vi "test.vi"() -> ()   [LabVIEW 2012]
uses:
  <vilib>/Platform/TimedLoop/XDataNode/timing_clust.ctl
  <vilib>/Platform/TimedLoop/XDataNode/nitl_modes.ctl
  <vilib>/Platform/TimedLoop/XDataNode/wakeup.ctl
  <vilib>/platform/TimedLoop/XDataNode/XDataNode.xnode
  <vilib>/Platform/TimedLoop/XDataNode/XDNodeRunTimeDep.lvlib
panel:
  out "CoolSnap Slave":bool
  out "Pixelfly Slave":bool
  out "ProEM Slave":bool
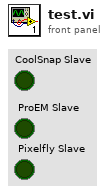
[diagram p1: front panel]
types:
  T1 = typedef "XDNodeRunTimeDep.lvlib/timing_clust.ctl" = cluster{"Expected End [f-1]":u64, "Actual End [f-1]":u64, "Finished Late? [f-1]":bool, "Expected End [i-1]":u64, "Actual End [i-1]":u64, "Finished Late? [i-1]":bool, "Expected Start [i]":u64, "Actual Start [i]":u64, "Expected Start [f]":u64, "Actual Start [f]":u64, "Source Name":string, "Structure Name":string, "Period":i64, "Deadline":i64, "Offset":i64, "Start":i64, "Priority":i32, "Timeout":i32, "Mode":T2, "Wakeup Reason":T3, "Error":errorcluster, "Source Type":string, "Secondary Source Type":string, "Global End Time":u64, "Global Start Time":u64, "Frame Duration":u64, "Iteration Duration":u64, "Assigned CPU":i32, "I/O Scan Engine Mode":u32}
  T2 = typedef "XDNodeRunTimeDep.lvlib/nitl_modes.ctl" = enum32{"No Change", "Process missed periods, maintain original phase", "Discard missed periods, maintain original phase", "Process missed periods, ignore original phase", "Discard missed periods, ignore original phase"}
  T3 = typedef "XDNodeRunTimeDep.lvlib/wakeup.ctl" = enum32{"Normal", "Aborted", "Asynchronous wakeup", "Timing source error", "Timed loop error", "Timeout"}
  T4 = typedef "LVDateTimeRec.ctl" = cluster{"fractional second":dbl, "second":i32, "minute":i32, "hour":i32, "day of month":i32, "month":i32, "year":i32, "day of week":i32, "day of year":i32, "DST":i32}
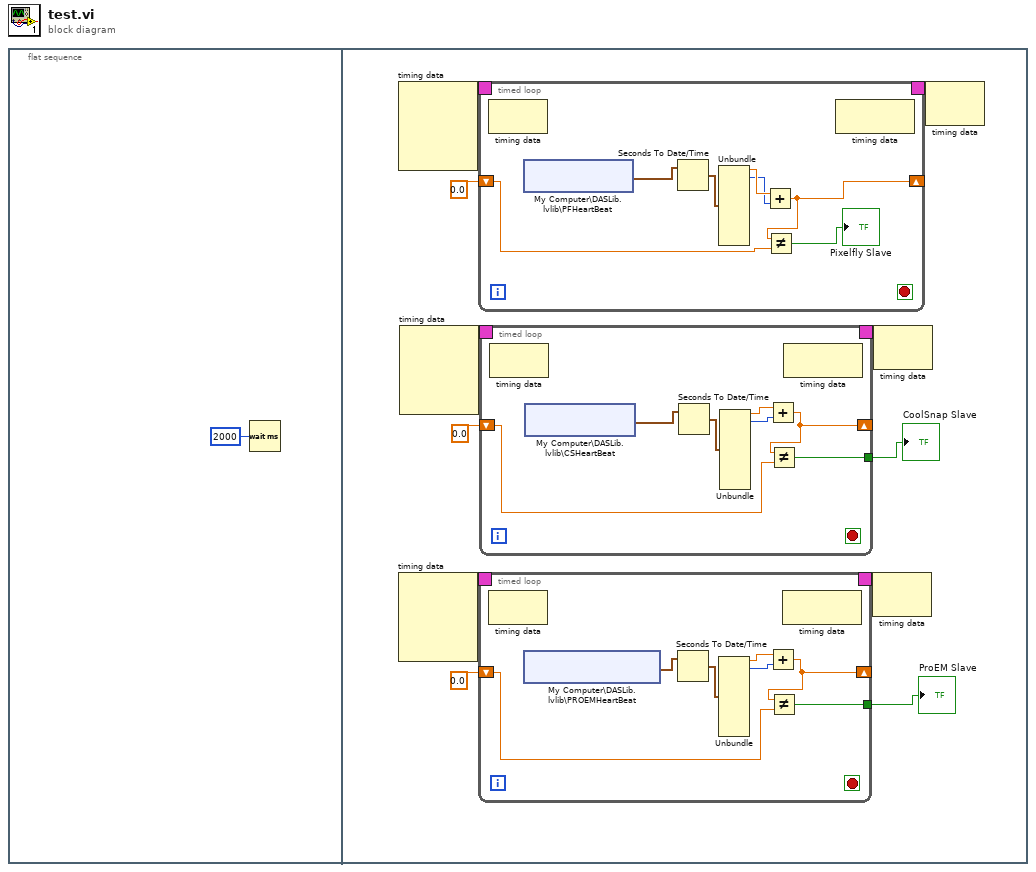
[diagram p0: block diagram]
diagram:
  n1 = flat-sequence {
    frame #0 {
      n2 = Wait (ms)(milliseconds to wait=u32 2000) -> ()  [unwired: 1 out]
    }
    frame #1 {
      n3 = node-c288() -> (w12:T1)  [unwired: 4 in]
      n4 = node-c288() -> (w8:T1)  [unwired: 4 in]
      n5 = node-c288() -> (w10:T1)  [unwired: 4 in]
      n6 = timed-loop {
        timing: w12 -> [_]
        timing-out: [_] -> w11
        shift-right: [w37] -> _
        shift-left: 0.0 ("fractional second") -> [w36]
        stop <- _ stop-if-true
        n7 = node-c288() -> ()  [unwired: 1 in, 1 out]
        n8 = shared-variable "My Computer\\DASLib.lvlib\\PFHeartBeat"() -> (w41:timestamp)  [unwired: 1 in, 2 out]
        n9 = Seconds To Date/Time(time stamp (now)=w41) -> (date time rec=w40:T4)  [unwired: 1 in]
        n10 = Unbundle(w40) -> ("fractional second"=w39:dbl, "second"=w38:i32)  [unwired: 8 out]
        n11 = Add(x=w39, y=w38) -> (x+y=w37:dbl)
        n12 = Not Equal?(x=w37, y=w36) -> (x != y?=→"Pixelfly Slave":bool)
        n13 = node-c288() -> ()  [unwired: 1 in, 1 out]
      }
      n14 = timed-loop {
        timing: w8 -> [_]
        timing-out: [_] -> w7
        shift-right: [w13] -> _
        shift-left: 0.0 ("fractional second") -> [w17]
        tunnel: [w16] -> w2
        stop <- _ stop-if-true
        n15 = node-c288() -> ()  [unwired: 1 in, 1 out]
        n16 = shared-variable "My Computer\\DASLib.lvlib\\PROEMHeartBeat"() -> (w19:timestamp)  [unwired: 1 in, 2 out]
        n17 = Seconds To Date/Time(time stamp (now)=w19) -> (date time rec=w18:T4)  [unwired: 1 in]
        n18 = Unbundle(w18) -> ("fractional second"=w15:dbl, "second"=w14:i32)  [unwired: 8 out]
        n19 = Add(x=w15, y=w14) -> (x+y=w13:dbl)
        n20 = Not Equal?(x=w13, y=w17) -> (x != y?=w16:bool)
        n21 = node-c288() -> ()  [unwired: 1 in, 1 out]
      }
      "ProEM Slave" <- w2
      n22 = timed-loop {
        timing: w10 -> [_]
        timing-out: [_] -> w9
        shift-right: [w24] -> _
        shift-left: 0.0 ("fractional second") -> [w25]
        tunnel: [w28] -> w3
        stop <- _ stop-if-true
        n23 = node-c288() -> ()  [unwired: 1 in, 1 out]
        n24 = shared-variable "My Computer\\DASLib.lvlib\\CSHeartBeat"() -> (w30:timestamp)  [unwired: 1 in, 2 out]
        n25 = Seconds To Date/Time(time stamp (now)=w30) -> (date time rec=w29:T4)  [unwired: 1 in]
        n26 = Unbundle(w29) -> ("fractional second"=w26:dbl, "second"=w27:i32)  [unwired: 8 out]
        n27 = Add(x=w26, y=w27) -> (x+y=w24:dbl)
        n28 = Not Equal?(x=w24, y=w25) -> (x != y?=w28:bool)
        n29 = node-c288() -> ()  [unwired: 1 in, 1 out]
      }
      "CoolSnap Slave" <- w3
      n30 = node-c288(w7) -> ()  [unwired: 1 out]
      n31 = node-c288(w9) -> ()  [unwired: 1 out]
      n32 = node-c288(w11) -> ()  [unwired: 1 out]
    }
  }
